vi "Main.vi"(11 "Module Admin":refnum<class "Delacor_lib_QMH_Module Admin.lvclass">) -> ()   [LabVIEW 2020, in "Settings.lvlib"]
doc: "This template is based off of the Queued Message Handler design pattern and the Queued Message Handler project template that ships with LabVIEW.\n\nThe main difference is that the queue is private to this module and communication between modules is performed via Broadcast and Request events.\n\nRequest events are wrapped in public API methods and are handled in the Event Handling Loop (EHL) of this VI. Any module can register for Broadcast events sent by this module. The EHL generates messages based on user interface actions.\n\nThe Message Handling Loop (MHL) processes messages generated by the EHL, or by other messages. The messages are string values, so new messages can be added easily to the Message Cases case structure in the MHL. Each message cluster can also provide an optional value for Message Data, which is a variant that can be converted to whatever message-specific data is required.\n_____\nBased on Delacor QMH Project Template 6.0.0.89."
uses:
  Settings.lvlib
  <vilib>/Delacor/Delacor QMH/Libraries/Module Admin_class/Delacor_lib_QMH_Module Admin.lvclass
  Acquisition/DigitalConfig--cluster.ctl
  Acquisition/AnalogConfig--cluster.ctl
  AcqType--enum.ctl
  TestName--control.ctl
  Module Data--cluster.ctl
  Stop Argument--cluster.ctl
  <vilib>/Delacor/Delacor QMH/Libraries/Message Queue_class/Delacor_lib_QMH_Message Queue.lvclass/Delacor_lib_QMH_Message Queue.ctl
  <vilib>/Delacor/Delacor QMH/Libraries/Module Admin_class/Delacor_lib_QMH_Module Admin.lvclass/Delacor_lib_QMH_Module Admin.ctl
  DeleteOneTask Argument--cluster.ctl
  DeleteAllTask Argument--cluster.ctl
  AddTask Argument--cluster.ctl
  Return Argument--cluster.ctl
  TestName Argument--cluster.ctl
  <vilib>/Utility/miscctls.llb/LVPointTypeDef.ctl
  <vilib>/Delacor/Delacor QMH/Libraries/Message Queue_class/Delacor_lib_QMH_Enqueue Message (Single).vi
  <vilib>/Delacor/Delacor QMH/Libraries/Module Admin_class/Delacor_lib_QMH_Get External Launch.vi
  <vilib>/Utility/error.llb/Error Cluster From Error Code.vi
  <vilib>/ErrorRing/Error Ring.xnode
  <vilib>/Delacor/Delacor QMH/Libraries/Message Queue_class/Delacor_lib_QMH_Message Queue.lvclass
  Acquisition/Acquisition.lvlib
panel:
  in  "DeleteAll":bool
  in  "Remove Button":bool
  in  "Add Button":bool
  in  "Regresar":bool
  in  "TestName":T1
  in  "AcquisitionType":T2
  in  "AnalogConfig":T3
  in  "DigitalConfig":T4
  out "error out":errorcluster
  out "Status":string
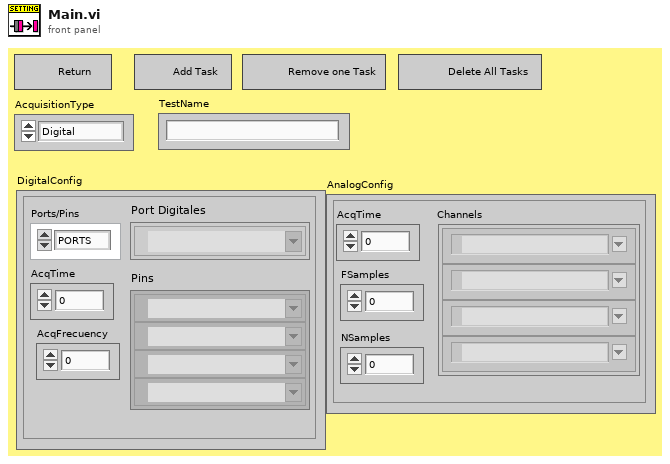
[diagram p1: front panel]
types:
  T1 = typedef "TestName--control.ctl" = string
  T2 = typedef "AcqType--enum.ctl" = enum16{"Digital", "Analog"}
  T3 = typedef "AnalogConfig--cluster.ctl" = cluster{"AcqTime":dbl, "FSamples":dbl, "NSamples":dbl, "Channels":tag[]}
  T4 = typedef "DigitalConfig--cluster.ctl" = cluster{"Ports/Pins":enum16{"PORTS", "PINS"}, "AcqTime":dbl, "AcqFrecuency":dbl, "Port Digitales":tag[], "Pins":tag[]}
  T5 = typedef "Acquisition.lvlib/Broadcast Events--cluster.ctl" = cluster{"Module Did Init":refnum<user-event>, "Status Updated":refnum<user-event>, "Error Reported":refnum<user-event>, "Module Did Stop":refnum<user-event>, "Update Module Execution Status":refnum<user-event>, "AnalogDataAcquired":refnum<user-event>, "DigitalDataAcquired":refnum<user-event>, "TypeAcq":refnum<user-event>}
  T6 = typedef "Settings.lvlib/Request Events--cluster.ctl" = cluster{"Stop Module":refnum<user-event>, "Show Panel":refnum<user-event>, "Hide Panel":refnum<user-event>, "Get Module Execution Status":refnum<user-event>, "Show Diagram":refnum<user-event>, "DeleteOneTask":refnum<user-event>, "DeleteAllTask":refnum<user-event>, "AddTask":refnum<user-event>, "Return":refnum<user-event>, "TestName":refnum<user-event>}
  T7 = typedef "Settings.lvlib/Module Data--cluster.ctl" = cluster{"Status":string, "AcquisitionType":T2, "AnalogConfig":T3, "DigitalConfig":T4, "TestName":T1}
  T8 = enum32{"invalid lock state", "Not Locked", "Locked (No Password)", "Password-protected"}
  T9 = typedef "Settings.lvlib/Stop Argument--cluster.ctl" = cluster{"Origin":string, "Exit via Stop Module Req?":bool, "Wait for Module to stop?":bool}
  T10 = typedef "Settings.lvlib/DeleteOneTask Argument--cluster.ctl" = cluster{"Boolean":bool}
  T11 = typedef "Settings.lvlib/DeleteAllTask Argument--cluster.ctl" = cluster{"Boolean":bool}
  T12 = typedef "Settings.lvlib/AddTask Argument--cluster.ctl" = cluster{"AcquisitionType":T2, "AnalogConfig":T3, "DigitalConfig":T4, "TestName":T1}
  T13 = typedef "Settings.lvlib/Return Argument--cluster.ctl" = cluster{"Boolean":bool}
  T14 = typedef "Settings.lvlib/TestName Argument--cluster.ctl" = cluster{"Name":string}
  T15 = typedef "LVPointTypeDef.ctl" = cluster{"Horizontal":i16, "Vertical":i16}
  T16 = enum32{"Invalid", "Standard", "Closed", "Hidden", "Minimized", "Maximized"}
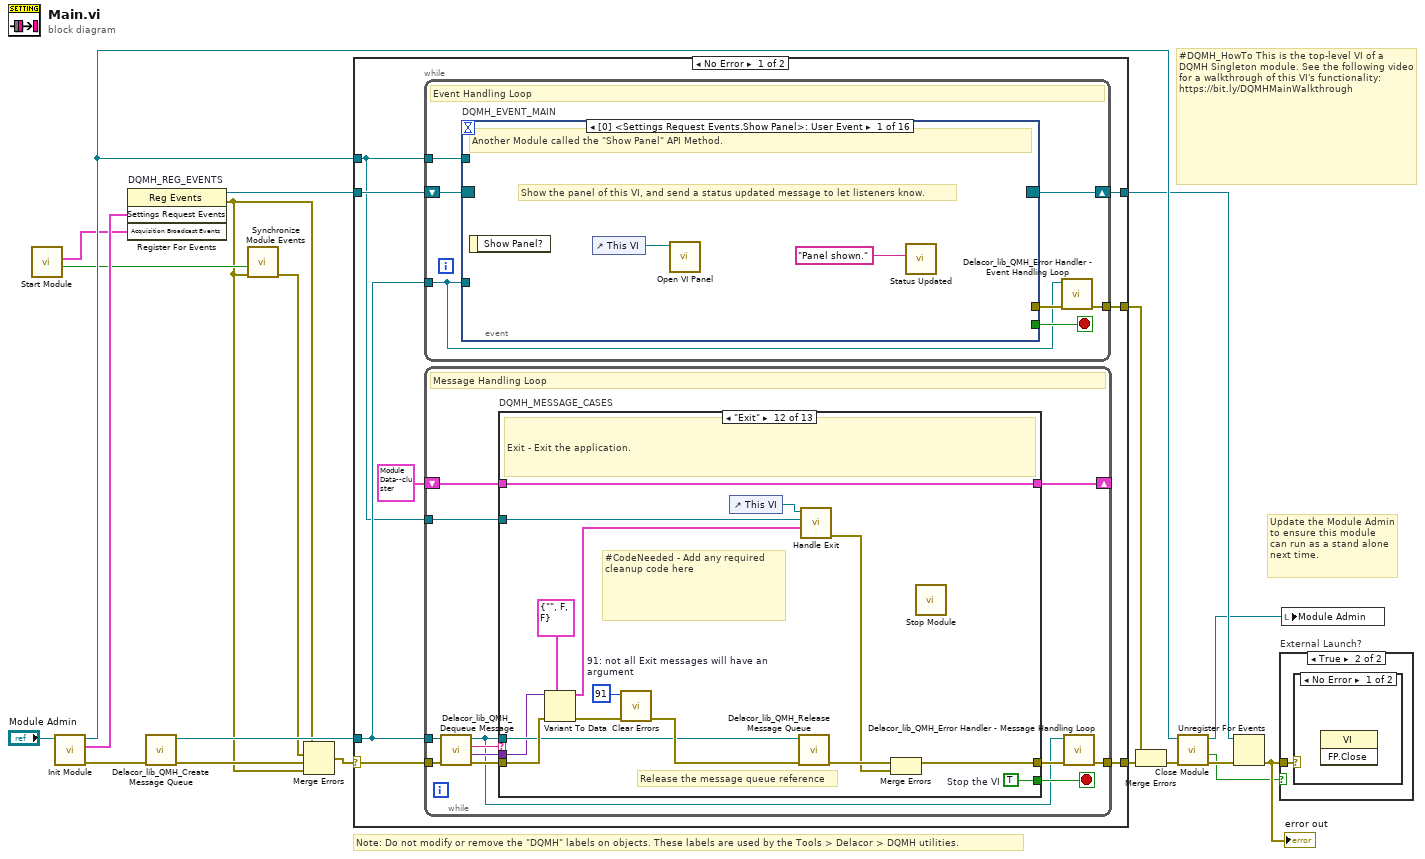
[diagram p0: block diagram]
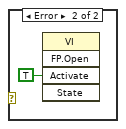
[diagram p3: hidden frame]
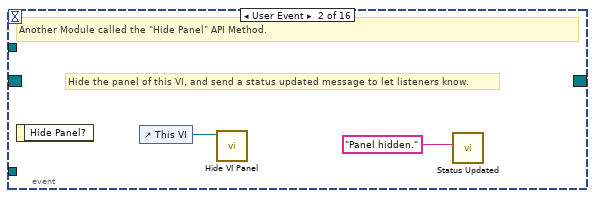
[diagram p4: hidden frame]
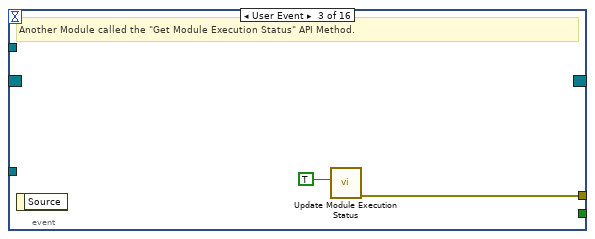
[diagram p5: hidden frame]
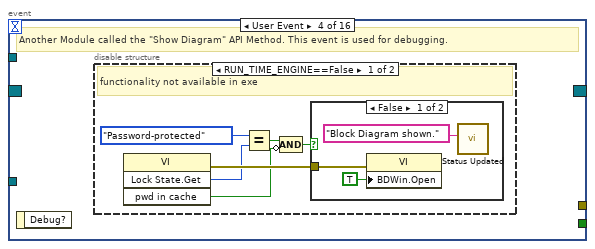
[diagram p6: hidden frame]
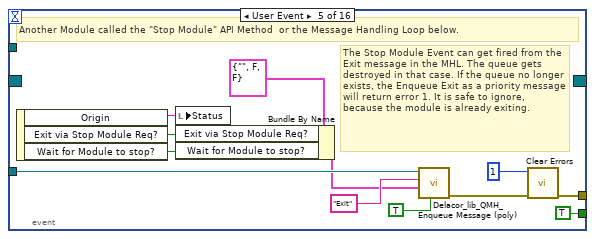
[diagram p9: hidden frame]
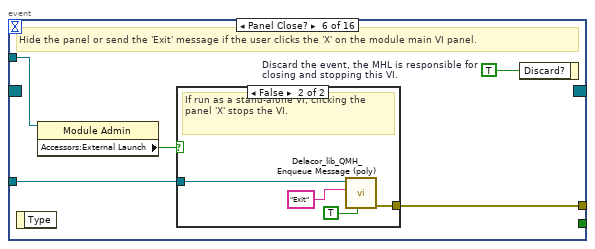
[diagram p10: hidden frame]
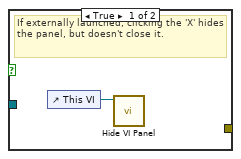
[diagram p11: hidden frame]
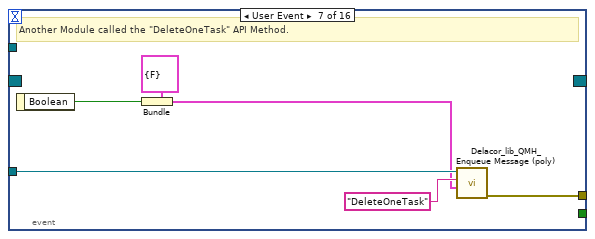
[diagram p12: hidden frame]
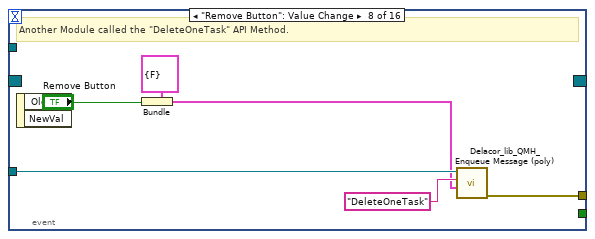
[diagram p13: hidden frame]
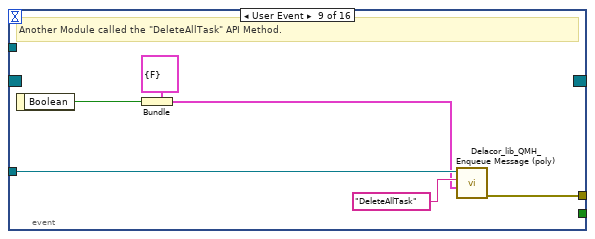
[diagram p14: hidden frame]
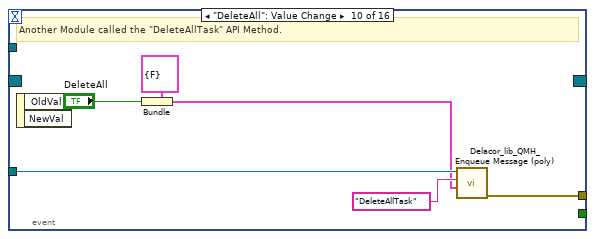
[diagram p15: hidden frame]
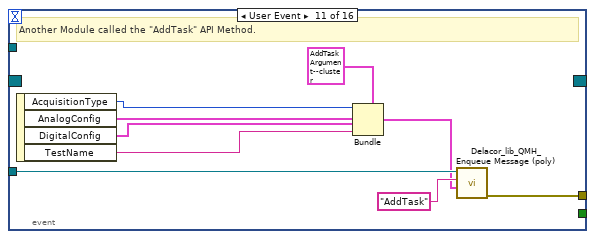
[diagram p16: hidden frame]
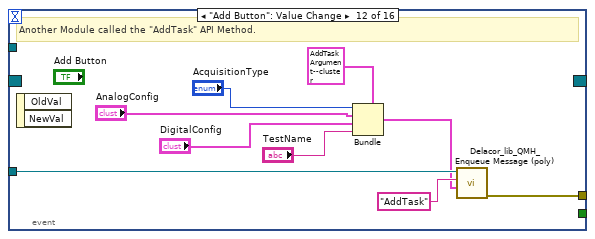
[diagram p17: hidden frame]
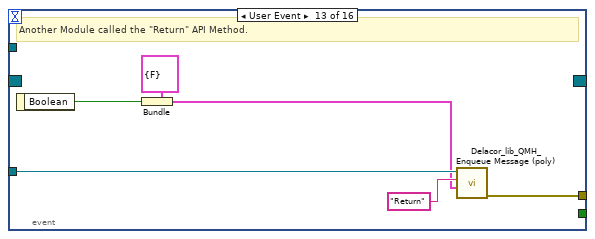
[diagram p18: hidden frame]
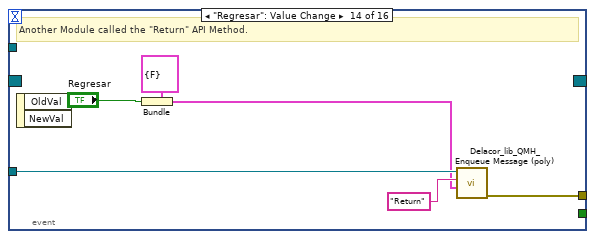
[diagram p19: hidden frame]
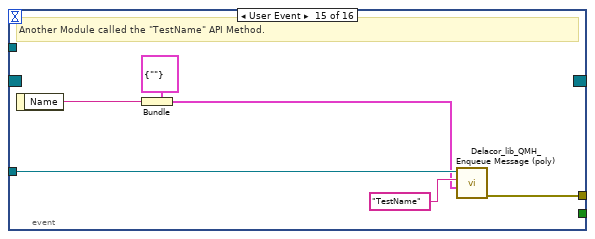
[diagram p20: hidden frame]
diagram:
  # "#DQMH_HowTo This is the top-level VI of a DQMH Singleton module. See the following video for a walkthrough of this VI's functionality: https://bit.ly/DQMHMainWalkthrough"
  # "Note: Do not modify or remove the \"DQMH\" labels on objects. These labels are used by the Tools > Delacor > DQMH utilities."
  # "Update the Module Admin to ensure this module can run as a stand alone next time."
  n1 = call "Start Module.vi"() -> ("Wait for Event Sync?"=w3:bool, "Acquisition Broadcast Events"=w4:T5)  [unwired: 8 in, 2 out]
  n2 = call "Init Module.vi"("Singleton Module Admin in"="Module Admin") -> ("error out"=w19:errorcluster, "Settings Request Events"=w9:T6, "Singleton Module Admin out"=w12:refnum<class "Delacor_lib_QMH_Module Admin.lvclass">)  [unwired: 8 in]
  n3 = register-events "DQMH_REG_EVENTS"(w9, w4) -> (reference out=w10:refnum<event-registration>, error out=w1:errorcluster)  [unwired: 2 in]
  n4 = call <vilib>:"Delacor_lib_QMH_Create Message Queue.vi"("error in"=w19) -> ("error out"=w14:errorcluster, "Message Queue"=w8:refnum<class "Delacor_lib_QMH_Message Queue.lvclass">)  [unwired: 9 in]
  n5 = call "Synchronize Module Events.vi"("error in"=w1, "Wait for Event Sync?"=w3) -> ("error out"=w2:errorcluster)  [unwired: 9 in]
  n6 = Merge Errors(w1, w2, w14, w1) -> (w13:errorcluster)
  n7 = case shown="No Error" w13 {
    selector: w13 -> [w26 w285]
    tunnel: [w28 w284] -> w20
    tunnel: [w25 w290] -> w11
    tunnel: w10 -> [w23 w290]
    tunnel: w8 -> [w22 w283]
    tunnel: [w27 _] -> w17
    tunnel: w12 -> [w21 w286]
    frame No Error {
      n8 = while {
        tunnel: w22 -> [w29]
        shift-right: [w32] -> w25
        shift-left: w23 -> [w33]
        tunnel: [w34] -> w27
        tunnel: w21 -> [w30]
        stop <- w31 stop-if-true
        # "Event Handling Loop"
        n9 = event "DQMH_EVENT_MAIN" shown="[0] <Settings Request Events.Show Panel>: User Event" {
          selector: w33 -> [_ _ _ _ _ _ _ _ _ _ _ _ _ _ _ _]
          dyn-events: [_ _ _ _ _ _ _ _ _ _ _ _ _ _ _ _] -> w32
          timeout: _ -> [_ _ _ _ _ _ _ _ _ _ _ _ _ _ _ _]
          tunnel: [_ _ _ _ TRUE ("Discard?") _ _ _ _ _ _ _ _ _ _ _] -> w31
          tunnel: w29 -> [_ _ _ _ w58 w65 w78 w84 w90 w96 w105 w114 w120 w126 w132 w138]
          tunnel: [_ _ w41 _ w61 w67 w73 w80 w85 w92 w101 w110 w115 w122 w127 w134] -> w35
          tunnel: w30 -> [_ _ _ _ _ w64 _ _ _ _ _ _ _ _ _ _]
          event User Event {
            # "Show the panel of this VI, and send a status updated message to let listeners know."
            # "Another Module called the \"Show Panel\" API Method."
            n10 = event-data() -> ()  [unwired: 1 in, 1 out]
            n11 = control-ref of="This VI"() -> (w37:refnum<vi>)
            n12 = call "Open VI Panel.vi"("VI"=w37) -> ()  [unwired: 10 in, 1 out]
            n13 = call "Status Updated.vi"("Status"="Panel shown." ("format string")) -> ()  [unwired: 10 in, 1 out]
          }
          event User Event {
            # "Hide the panel of this VI, and send a status updated message to let listeners know."
            # "Another Module called the \"Hide Panel\" API Method."
            n14 = event-data() -> ()  [unwired: 1 in, 1 out]
            n15 = control-ref of="This VI"() -> (w39:refnum<vi>)
            n16 = call "Hide VI Panel.vi"("VI"=w39) -> ()  [unwired: 10 in, 1 out]
            n17 = call "Status Updated.vi"("Status"="Panel hidden." ("format string")) -> ()  [unwired: 10 in, 1 out]
          }
          event User Event {
            # "Another Module called the \"Get Module Execution Status\" API Method."
            n18 = event-data() -> ()  [unwired: 1 in, 1 out]
            n19 = call "Update Module Execution Status.vi"("Running?"=TRUE) -> ("error out"=w41:errorcluster)  [unwired: 10 in]
          }
          event User Event {
            # "Another Module called the \"Show Diagram\" API Method. This event is used for debugging."
            n20 = event-data() -> ()  [unwired: 1 in, 1 out]
            n21 = disable-structure shown="RUN_TIME_ENGINE==False" {
              frame condition #0 (active) {
                # "functionality not available in exe"
                n22 = invoke class="VI" method="Lock State.Get"() -> (error out=w47:errorcluster, "Get Lock State"=w46:T8, "pwd in cache"=w43:bool)  [unwired: 4 in, 1 out]
                n23 = Equal?(x=T8."Password-protected", y=w46) -> (x = y?=w44:bool)
                n24 = Compound Arithmetic op=AND(w44, invert w43) -> (w42:bool)
                n25 = case shown="False" w42 {
                  tunnel: w47 -> [w50 _]
                  frame False {
                    n26 = property class="VI"(error in=w50, "BDWin.Open"=TRUE ("Block Diagram Window:Open")) -> ()  [unwired: 1 in, 2 out]
                    n27 = call "Status Updated.vi"("Status"="Block Diagram shown." ("format string")) -> ()  [unwired: 10 in, 1 out]
                  }
                  frame True {
                    # "Password-protected VI, and the password is not in the cache. Do not show the diagram."
                  }
                }
              }
              frame condition #1 {
              }
            }
          }
          event User Event {
            # "The Stop Module Event can get fired from the Exit message in the MHL. The queue gets destroyed in that case. If the queue no longer exists, the Enqueue Exit as a priority message will return error 1. It is safe to ignore, because the module is already exiting."
            # "Another Module called the \"Stop Module\" API Method  or the Message Handling Loop below."
            n28 = event-data() -> ("Origin"=w57:string, "Exit via Stop Module Req?"=w53:bool, "Wait for Module to stop?"=w52:bool)  [unwired: 1 in]
            n29 = local write "Status"(w57) -> ()
            n30 = Bundle By Name(cluster=T9 {"Origin"="", "Exit via Stop Module Req?"=FALSE, "Wait for Module to stop?"=FALSE} ("Stop Argument"), "Exit via Stop Module Req?"=w53, "Wait for Module to stop?"=w52) -> (w51:T9)
            n31 = call-poly <vilib>:"Delacor_lib_QMH_Enqueue Message (poly).vi"("Priority Message? (F)"=TRUE, "Message Data"=w51, "Message"="Exit", "Message Queue in"=w58) -> ("error out"=w62:errorcluster)  [unwired: 6 in, 1 out]
            n32 = call <vilib>:"Clear Errors.vi"("error in (no error)"=w62, "specific error code to clear (0: all)"=1) -> ("error out"=w61:errorcluster)  [unwired: 4 in, 1 out]
          }
          event Panel Close? {
            w66 = TRUE  # Discard the event, the MHL is responsible for closing and stopping this VI.
            # "Hide the panel or send the 'Exit' message if the user clicks the 'X' on the module main VI panel."
            n33 = event-data() -> ()  [unwired: 1 in, 1 out]
            n34 = property class="Module Admin"(reference=w64) -> ("Accessors:External Launch"=w63:bool)  [unwired: 1 in, 2 out]
            n35 = case shown="False" w63 {
              tunnel: w65 -> [_ w71]
              tunnel: [_ w72] -> w67
              frame True {
                # "If externally launched, clicking the 'X' hides the panel, but doesn't close it."
                n36 = control-ref of="This VI"() -> (w68:refnum<vi>)
                n37 = call "Hide VI Panel.vi"("VI"=w68) -> ()  [unwired: 10 in, 1 out]
              }
              frame False {
                # "If run as a stand-alone VI, clicking the panel 'X' stops the VI."
                n38 = call-poly <vilib>:"Delacor_lib_QMH_Enqueue Message (poly).vi"("Priority Message? (F)"=TRUE, "Message"="Exit", "Message Queue in"=w71) -> ("error out"=w72:errorcluster)  [unwired: 7 in, 1 out]
              }
            }
            n39 = event-data("Discard?"=w66) -> ()  [unwired: 1 in, 1 out]
          }
          event User Event {
            # "Another Module called the \"DeleteOneTask\" API Method."
            n40 = event-data() -> ("Boolean"=w74:bool)  [unwired: 1 in]
            n41 = Bundle(cluster=T10 {"Boolean"=FALSE} ("DeleteOneTask Argument"), "Boolean"=w74) -> (w75:T10)
            n42 = call-poly <vilib>:"Delacor_lib_QMH_Enqueue Message (poly).vi"("Message Data"=w75, "Message"="DeleteOneTask", "Message Queue in"=w78) -> ("error out"=w73:errorcluster)  [unwired: 7 in, 1 out]
          }
          event "Remove Button": Value Change {
            # "Another Module called the \"DeleteOneTask\" API Method."
            n43 = event-data() -> ()  [unwired: 1 in, 2 out]
            n44 = Bundle(cluster=T10 {"Boolean"=FALSE} ("DeleteOneTask Argument"), "Boolean"="Remove Button") -> (w81:T10)
            n45 = call-poly <vilib>:"Delacor_lib_QMH_Enqueue Message (poly).vi"("Message Data"=w81, "Message"="DeleteOneTask", "Message Queue in"=w84) -> ("error out"=w80:errorcluster)  [unwired: 7 in, 1 out]
          }
          event User Event {
            # "Another Module called the \"DeleteAllTask\" API Method."
            n46 = event-data() -> ("Boolean"=w86:bool)  [unwired: 1 in]
            n47 = Bundle(cluster=T11 {"Boolean"=FALSE} ("DeleteAllTask Argument"), "Boolean"=w86) -> (w87:T11)
            n48 = call-poly <vilib>:"Delacor_lib_QMH_Enqueue Message (poly).vi"("Message Data"=w87, "Message"="DeleteAllTask", "Message Queue in"=w90) -> ("error out"=w85:errorcluster)  [unwired: 7 in, 1 out]
          }
          event "DeleteAll": Value Change {
            # "Another Module called the \"DeleteAllTask\" API Method."
            n49 = event-data() -> ()  [unwired: 1 in, 2 out]
            n50 = Bundle(cluster=T11 {"Boolean"=FALSE} ("DeleteAllTask Argument"), "Boolean"="DeleteAll") -> (w93:T11)
            n51 = call-poly <vilib>:"Delacor_lib_QMH_Enqueue Message (poly).vi"("Message Data"=w93, "Message"="DeleteAllTask", "Message Queue in"=w96) -> ("error out"=w92:errorcluster)  [unwired: 7 in, 1 out]
          }
          event User Event {
            # "Another Module called the \"AddTask\" API Method."
            n52 = event-data() -> ("AcquisitionType"=w100:T2, "AnalogConfig"=w99:T3, "DigitalConfig"=w98:T4, "TestName"=w97:T1)  [unwired: 1 in]
            n53 = Bundle(cluster=T12 {"AcquisitionType"=enum."Digital", "AnalogConfig"={"AcqTime"=0.0, "FSamples"=0.0, "NSamples"=0.0, "Channels"=[]}, "DigitalConfig"={"Ports/Pins"=enum."PORTS", "AcqTime"=0.0, "AcqFrecuency"=0.0, "Port Digitales"=[], "Pins"=[]}, "TestName"=""} ("AddTask Argument"), "AcquisitionType"=w100, "AnalogConfig"=w99, "DigitalConfig"=w98, "TestName"=w97) -> (w102:T12)
            n54 = call-poly <vilib>:"Delacor_lib_QMH_Enqueue Message (poly).vi"("Message Data"=w102, "Message"="AddTask", "Message Queue in"=w105) -> ("error out"=w101:errorcluster)  [unwired: 7 in, 1 out]
          }
          event "Add Button": Value Change {
            # "Another Module called the \"AddTask\" API Method."
            n55 = event-data() -> ()  [unwired: 1 in, 2 out]
            n56 = Bundle(cluster=T12 {"AcquisitionType"=enum."Digital", "AnalogConfig"={"AcqTime"=0.0, "FSamples"=0.0, "NSamples"=0.0, "Channels"=[]}, "DigitalConfig"={"Ports/Pins"=enum."PORTS", "AcqTime"=0.0, "AcqFrecuency"=0.0, "Port Digitales"=[], "Pins"=[]}, "TestName"=""} ("AddTask Argument"), "AcquisitionType"="AcquisitionType", "AnalogConfig"="AnalogConfig", "DigitalConfig"="DigitalConfig", "TestName"="TestName") -> (w111:T12)
            n57 = call-poly <vilib>:"Delacor_lib_QMH_Enqueue Message (poly).vi"("Message Data"=w111, "Message"="AddTask", "Message Queue in"=w114) -> ("error out"=w110:errorcluster)  [unwired: 7 in, 1 out]
          }
          event User Event {
            # "Another Module called the \"Return\" API Method."
            n58 = event-data() -> ("Boolean"=w116:bool)  [unwired: 1 in]
            n59 = Bundle(cluster=T13 {"Boolean"=FALSE} ("Return Argument"), "Boolean"=w116) -> (w117:T13)
            n60 = call-poly <vilib>:"Delacor_lib_QMH_Enqueue Message (poly).vi"("Message Data"=w117, "Message"="Return", "Message Queue in"=w120) -> ("error out"=w115:errorcluster)  [unwired: 7 in, 1 out]
          }
          event "Regresar": Value Change {
            # "Another Module called the \"Return\" API Method."
            n61 = event-data() -> ()  [unwired: 1 in, 2 out]
            n62 = Bundle(cluster=T13 {"Boolean"=FALSE} ("Return Argument"), "Boolean"="Regresar") -> (w123:T13)
            n63 = call-poly <vilib>:"Delacor_lib_QMH_Enqueue Message (poly).vi"("Message Data"=w123, "Message"="Return", "Message Queue in"=w126) -> ("error out"=w122:errorcluster)  [unwired: 7 in, 1 out]
          }
          event User Event {
            # "Another Module called the \"TestName\" API Method."
            n64 = event-data() -> ("Name"=w128:string)  [unwired: 1 in]
            n65 = Bundle(cluster=T14 {"Name"=""} ("TestName Argument"), "Name"=w128) -> (w129:T14)
            n66 = call-poly <vilib>:"Delacor_lib_QMH_Enqueue Message (poly).vi"("Message Data"=w129, "Message"="TestName", "Message Queue in"=w132) -> ("error out"=w127:errorcluster)  [unwired: 7 in, 1 out]
          }
          event Value Change {
            # "Another Module called the \"TestName\" API Method."
            n67 = event-data() -> ()  [unwired: 1 in, 2 out]
            n68 = local read "TestName"() -> (w133:T1)
            n69 = Bundle(cluster=T14 {"Name"=""} ("TestName Argument"), "Name"=w133) -> (w135:T14)
            n70 = call-poly <vilib>:"Delacor_lib_QMH_Enqueue Message (poly).vi"("Message Data"=w135, "Message"="TestName", "Message Queue in"=w138) -> ("error out"=w134:errorcluster)  [unwired: 7 in, 1 out]
          }
        }
        n71 = call-dynamic "Delacor_lib_QMH_Error Handler - Event Handling Loop.vi"("error in"=w35, "Message Queue in"=w29) -> ("dup error in"=w34:errorcluster)  [unwired: 8 in, 1 out]
      }
      n72 = while {
        tunnel: w22 -> [w141]
        shift-right: [w145] -> _
        shift-left: T7 {"Status"="", "AcquisitionType"=enum."Digital", "AnalogConfig"={"AcqTime"=0.0, "FSamples"=0.0, "NSamples"=0.0, "Channels"=[]}, "DigitalConfig"={"Ports/Pins"=enum."PORTS", "AcqTime"=0.0, "AcqFrecuency"=0.0, "Port Digitales"=[], "Pins"=[]}, "TestName"=""} ("Data Cluster") -> [w146]
        tunnel: w26 -> [w149]
        tunnel: [w147] -> w28
        tunnel: w21 -> [w139]
        stop <- w144 stop-if-true
        # "Message Handling Loop"
        n73 = call-dynamic "Delacor_lib_QMH_Dequeue Message.vi"("error in"=w149, "Message Queue in"=w141) -> ("error out"=w148:errorcluster, "Message Data"=w142:variant, "Message"=w143:string, "Message Queue out"=w140:refnum<class "Delacor_lib_QMH_Message Queue.lvclass">)  [unwired: 6 in]
        n74 = case "DQMH_MESSAGE_CASES" shown="\"Exit\"" w143 {
          selector: w143 -> [_ _ _ _ _ _ _ _ _ _ _ _ w270]
          tunnel: w140 -> [_ _ _ _ _ w208 w218 _ _ _ w240 w262 _]
          tunnel: w148 -> [w175 w179 w186 w193 w204 w216 w227 w232 w235 w237 w247 w268 w272]
          tunnel: [w174 w179 w180 w187 w203 w210 w220 w232 w234 w237 w243 w265 w273] -> w150
          tunnel: w146 -> [w165 w178 w185 w192 w199 w215 w226 w231 w233 w236 w242 w261 w271]
          tunnel: [w164 w178 w185 w192 w198 w215 w222 w231 w233 w236 w242 w261 w271] -> w145
          tunnel: [_ _ _ _ _ _ _ _ _ _ _ w260 _] -> w144
          tunnel: w142 -> [_ _ w184 w191 w202 w214 w225 _ _ _ w241 w259 _]
          tunnel: w139 -> [w166 _ _ _ _ _ _ _ _ _ w239 w254 _]
          frame "Initialize" {
            w160 = "Initial Message" ("Initial Message")
            # "Crea la tabla y lee la ultima configuracion\nAdemas manda la secuencia a acquisition"
            # "Initialize - Any operation that needs to be done before the module can receive messages. Synchronize Caller Events.vi will inform Start Module.vi that the module has launched and is ready to receive messages. Module Did Init.vi will broadcast that the module initialized."
            n75 = call "Synchronize Caller Events.vi"("error in (no error)"=w175, "Singleton Module Admin in"=w166) -> ("error out"=w158:errorcluster, "Singleton Module Admin out"=w161:refnum<class "Delacor_lib_QMH_Module Admin.lvclass">)  [unwired: 8 in]
            n76 = call "READDB.vi"() -> ("Datos"=w151:string[][], "Max ID"=w152:i32)  [unwired: 8 in, 2 out]
            n77 = property class="Module Admin"(reference=w161) -> ("Accessors:External Launch"=w170:bool)  [unwired: 1 in, 2 out]
            n78 = call "Set Secuence.vi"("Secuence"=w151, "ID Max"=w152) -> ()  [unwired: 9 in, 1 out]
            n79 = call "CreateTableDB.vi"("error in (no error)"=w158) -> ("error out"=w157:errorcluster)  [unwired: 10 in]
            n80 = call "Module Name--constant.vi"() -> ("Module Name"=w173:string)  [unwired: 11 in]
            n81 = call "ReadConfig.vi"("error in (no error)"=w157) -> ("error out"=w156:errorcluster, "AcquisitionType"=w155:T2, "AnalogOut"=w154:T3, "DigitalOut"=w153:T4)  [unwired: 7 in]
            n82 = Select(t=T16."Hidden" ("State"), s=w170, f=T16."Standard" ("State")) -> (s? t:f=w167:T16)
            n83 = property class="VI"("Front Panel.Title"=w173) -> (reference out=w172:refnum<vi>, error out=w177:errorcluster)  [unwired: 2 in]
            n84 = invoke class="VI" method="FP.Open"(reference=w172, error in=w177, "State"=w167) -> (reference out=w171:refnum<vi>, error out=w176:errorcluster)  [unwired: 2 in, 3 out]
            n85 = local write "DigitalConfig"(w153) -> ()
            n86 = local write "AnalogConfig"(w154) -> ()
            n87 = local write "AcquisitionType"(w155) -> ()
            n88 = call "Module Name--constant.vi"() -> ("Module Name"=w162:string)  [unwired: 11 in]
            n89 = invoke class="VI" method="FP.Center"(reference=w171, error in=w176) -> ()  [unwired: 1 in, 3 out]
            n90 = call "Module Did Init.vi"("error in (no error)"=w156, "Initialized?"=TRUE, "Origin"=w162) -> ("error out"=w174:errorcluster)  [unwired: 8 in]
            n91 = Bundle By Name(cluster=w165, "Status"=w160) -> (w164:T7)
            n92 = property on="Pane" class="Pane"("Origin"=T15 {"Horizontal"=0, "Vertical"=0}) -> ()  [unwired: 2 in, 2 out]
            "Status" <- w160
          }
          frame "---Module Specific---" {
            # "Separator -- The following cases handle messages specific to this Module."
          }
          frame "DeleteOneTask" {
            # "Borra la ultima tarea"
            n93 = Variant To Data(error in=w186, type=T10 {"Boolean"=FALSE} ("DeleteOneTask Argument"), Variant=w184) -> (data=w182:T10, error out=w181:errorcluster)
            n94 = Unbundle By Name(w182) -> ()  [unwired: 1 out]
            n95 = call "DeleteONE.vi"("error in (no error)"=w181) -> ("error out"=w180:errorcluster)  [unwired: 10 in]
          }
          frame "DeleteAllTask" {
            # "Borra todas las tareas"
            n96 = Variant To Data(error in=w193, type=T11 {"Boolean"=FALSE} ("DeleteAllTask Argument"), Variant=w191) -> (data=w189:T11, error out=w188:errorcluster)
            n97 = Unbundle By Name(w189) -> ()  [unwired: 1 out]
            n98 = call "DeleteALL.vi"("error in (no error)"=w188) -> ("error out"=w187:errorcluster)  [unwired: 10 in]
          }
          frame "AddTask" {
            # "Agrega la tarea"
            n99 = Variant To Data(error in=w204, type=T12 {"AcquisitionType"=enum."Digital", "AnalogConfig"={"AcqTime"=0.0, "FSamples"=0.0, "NSamples"=0.0, "Channels"=[]}, "DigitalConfig"={"Ports/Pins"=enum."PORTS", "AcqTime"=0.0, "AcqFrecuency"=0.0, "Port Digitales"=[], "Pins"=[]}, "TestName"=""} ("AddTask Argument"), Variant=w202) -> (data=w200:T12, error out=w203:errorcluster)
            n100 = Unbundle By Name(w200) -> ("TestName"=w195:T1, "AcquisitionType"=w194:T2, "DigitalConfig"=w196:T4, "AnalogConfig"=w197:T3)
            n101 = call "NameTest.vi"("String"=w195) -> ()  [unwired: 10 in, 1 out]
            n102 = call "TypeSignal.vi"("SygnalType"=w194) -> ()  [unwired: 10 in, 1 out]
            n103 = Bundle By Name(cluster=w199, "TestName"=w195) -> (w198:T7)
            n104 = case shown="\"Digital\", Default" w194 {
              tunnel: w197 -> [_ w206]
              tunnel: w196 -> [w205 _]
              frame "Digital", Default {
                n105 = call "DigitalConfigWrite.vi"("DigitalConfig"=w205) -> ()  [unwired: 10 in, 1 out]
              }
              frame "Analog" {
                n106 = call "AnalogConfigWrite.vi"("AnalogConfig"=w206) -> ()  [unwired: 10 in, 1 out]
              }
            }
          }
          frame "Return" {
            # "Regresa al UI"
            n107 = Variant To Data(error in=w216, type=T13 {"Boolean"=FALSE} ("Return Argument"), Variant=w214) -> (data=w212:T13, error out=w211:errorcluster)
            n108 = Unbundle By Name(w212) -> ()  [unwired: 1 out]
            n109 = call "Hide Panel.vi"("error in (no error)"=w211) -> ("error out"=w209:errorcluster)  [unwired: 10 in]
            n110 = call-poly <vilib>:"Delacor_lib_QMH_Enqueue Message (poly).vi"("error in"=w209, "Message"="Sent", "Message Queue in"=w208) -> ("error out"=w210:errorcluster)  [unwired: 7 in, 1 out]
          }
          frame "TestName" {
            # "Adquiere el valor del nombre de la prueba"
            n111 = Variant To Data(error in=w227, type=T14 {"Name"=""} ("TestName Argument"), Variant=w225) -> (data=w223:T14, error out=w219:errorcluster)
            n112 = Unbundle By Name(w223) -> ("Name"=w221:string)
            n113 = Bundle By Name(cluster=w226, "TestName"=w221) -> (w222:T7)
            n114 = call-poly <vilib>:"Delacor_lib_QMH_Enqueue Message (poly).vi"("error in"=w219, "Message"="Sent", "Message Queue in"=w218) -> ("error out"=w220:errorcluster)  [unwired: 7 in, 1 out]
          }
          frame "Sent" {
            # "Request para mandar la secuencia a adquisicion"
            # "Guardo el nombre de la prueba"
            n115 = Unbundle By Name(w231) -> ("TestName"=w230:T1)
            n116 = call "READDB.vi"() -> ("Datos"=w228:string[][], "Max ID"=w229:i32)  [unwired: 8 in, 2 out]
            n117 = call "Set Secuence.vi"("Secuence"=w228, "ID Max"=w229) -> ()  [unwired: 9 in, 1 out]
            n118 = call "NameTest.vi"("String"=w230) -> ()  [unwired: 10 in, 1 out]
          }
          frame "---Copy This Frame---" {
            # "Duplicate this frame when creating new messages.  Change this comment in the duplicated frame to describe this message."
            n119 = Merge Errors(w235) -> (w234:errorcluster)
          }
          frame "---Exit and Error Handling---" {
            # "Separator - The following cases handle errors and exit messages."
          }
          frame "Error" {
            # "#CodeRecommended - If you ever change the name of this \"Error\" message, you'll need to update the name in the Check Loop Error.vi as well."
            # "#CodeRecommended - If the module is running in standalone mode (External Launch = FALSE), this code will pop up an error dialog and call the 'Exit' message if an error occurs. Add more fine-grained error handling here."
            # "Error - Check the error message data and respond accordingly. This message is sent by the \"Error Handler\" VIs at the end of each loop in this application."
            n120 = property class="Module Admin"(reference=w239) -> ("Accessors:External Launch"=w238:bool)  [unwired: 1 in, 2 out]
            n121 = Variant To Data(error in=w247, type=errorcluster {"status"=FALSE, "code"=0, "source"=""} ("error constant"), Variant=w241) -> (data=w248:errorcluster, error out=w245:errorcluster)
            n122 = call "Error Reported.vi"("Error"=w248) -> ()  [unwired: 10 in, 1 out]
            n123 = case shown="False" w238 {
              tunnel: [w253 _] -> w244
              tunnel: w240 -> [w251 _]
              tunnel: w248 -> [w252 _]
              frame False {
                # "If the module is running standalone, then pop up an error dialog and call the \"Exit\" message."
                n124 = call <vilib>:"Simple Error Handler.vi"("error in (no error)"=w252) -> ()  [unwired: 4 in, 5 out]
                n125 = call-poly <vilib>:"Delacor_lib_QMH_Enqueue Message (poly).vi"("Priority Message? (F)"=TRUE, "Message"="Exit", "Message Queue in"=w251) -> ("error out"=w253:errorcluster)  [unwired: 7 in, 1 out]
              }
              frame True {
                # "If the module was launched externally, calling the Error Reported broadcast VI is the only action performed by the \"Error\" message. The module's caller can then process the error appropriately."
              }
            }
            n126 = Merge Errors(w245, w244) -> (w243:errorcluster)
            n127 = local write "error out"(w243) -> ()
          }
          frame "Exit" {
            w258 = 91  # 91: not all Exit messages will have an argument
            w260 = TRUE  # Stop the VI
            # "Release the message queue reference"
            # "#CodeNeeded - Add any required cleanup code here"
            # "Exit - Exit the application."
            n128 = Variant To Data(error in=w268, type=T9 {"Origin"="", "Exit via Stop Module Req?"=FALSE, "Wait for Module to stop?"=FALSE} ("Stop Argument"), Variant=w259) -> (data=w256:T9, error out=w264:errorcluster)
            n129 = call <vilib>:"Clear Errors.vi"("error in (no error)"=w264, "specific error code to clear (0: all)"=w258) -> ("error out"=w267:errorcluster)  [unwired: 4 in, 1 out]
            n130 = control-ref of="This VI"() -> (w255:refnum<vi>)
            n131 = call-dynamic "Delacor_lib_QMH_Release Message Queue.vi"("error in"=w267, "Message Queue"=w262) -> ("error out"=w266:errorcluster)  [unwired: 9 in]
            n132 = call "Handle Exit.vi"("Stop Argument"=w256, "Admin in"=w254, "VI reference"=w255) -> ("error out"=w263:errorcluster)  [unwired: 7 in, 1 out]
            n133 = Merge Errors(w266, w263) -> (w265:errorcluster)
            n134 = call "Stop Module.vi"() -> ()  [unwired: 11 in, 1 out]
          }
          frame Default {
            # "'Default' case only runs if there is a message that isn't defined in any of the other cases.  Output a programming error."
            n135 = call "Module Name--constant.vi"() -> ("Module Name"=w269:string)  [unwired: 11 in]
            n136 = xnode "Error Ring"("parameter 0"=w270, "parameter 1"=w269) -> ("error out"=w274:errorcluster)
            n137 = Merge Errors(w272, w274) -> (w273:errorcluster)
          }
        }
        n138 = call-dynamic "Delacor_lib_QMH_Error Handler - Message Handling Loop.vi"("error in"=w150, "Message Queue in"=w140) -> ("dup error in"=w147:errorcluster)  [unwired: 8 in, 1 out]
      }
    }
    frame Error {
      # "Synchronize Caller Events.vi will inform Start Module.vi that the module has launched and will let the code calling Start Module.vi register for broadcasts and would permit the caller receive the broadcast that an error occurred at launch time."
      n139 = call-dynamic "Delacor_lib_QMH_Release Message Queue.vi"("error in"=w285, "Message Queue"=w283) -> ("error out"=w284:errorcluster)  [unwired: 9 in]
      n140 = call "Synchronize Caller Events.vi"("Singleton Module Admin in"=w286) -> ("error out"=w291:errorcluster)  [unwired: 9 in, 1 out]
      n141 = call "Module Name--constant.vi"() -> ("Module Name"=w289:string)  [unwired: 11 in]
      n142 = Format Into String(format string="An error occurred during initialization. %s is no longer running.", w289) -> (resulting string=w287:string)  [unwired: 2 in, 1 out]
      n143 = Merge Errors(w284, w291) -> (w292:errorcluster)
      n144 = call "Stop Module.vi"() -> ()  [unwired: 11 in, 1 out]
      n145 = call "Error Reported.vi"("Additional Information"=w287, "Error"=w292) -> ()  [unwired: 9 in, 1 out]
    }
  }
  n146 = Merge Errors(w17, w20) -> (w16:errorcluster)
  n147 = call "Close Module.vi"("error in (no error)"=w16, "Module Admin in"=w12) -> ("error out"=w18:errorcluster, "External Launch"=w5:bool, "Module Admin out"=w6:refnum<class "Delacor_lib_QMH_Module Admin.lvclass">)  [unwired: 7 in]
  n148 = Unregister For Events(event registration refnum=w11, error in=w18) -> (error out=w15:errorcluster)
  "error out" <- w15
  n149 = case "External Launch?" shown="True" w5 {
    tunnel: w15 -> [_ w293]
    frame False {
    }
    frame True {
      n150 = case shown="No Error" w293 {
        frame No Error {
          n151 = invoke class="VI" method="FP.Close"() -> ()  [unwired: 3 in, 3 out]
        }
        frame Error {
          n152 = invoke class="VI" method="FP.Open"("Activate"=TRUE ("Activate?")) -> ()  [unwired: 4 in, 5 out]
        }
      }
    }
  }
  n153 = local write "Module Admin"(w6) -> ()
